vi "Select File.vi"(5 "PREV":bool, 6 "t in":i32, 7 "Bool Refnum in":refnum<vi>, 8 "error in (no error)":errorcluster, 9 "NEXT":bool, 10 "Bool Refnum 3":refnum<vi>, 11 "Boolean in":refnum<vi>) -> (0 "error out":errorcluster, 3 "t out":i32)   [LabVIEW 2020]
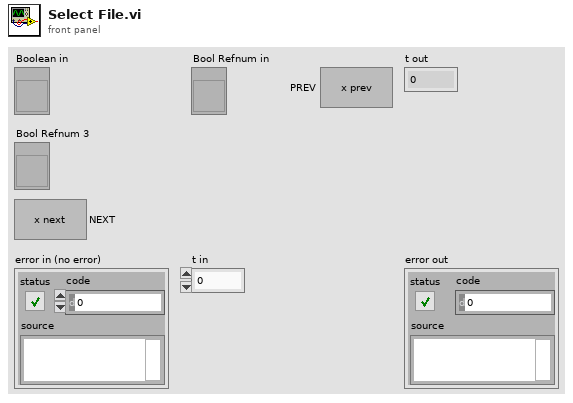
[diagram p1: front panel]
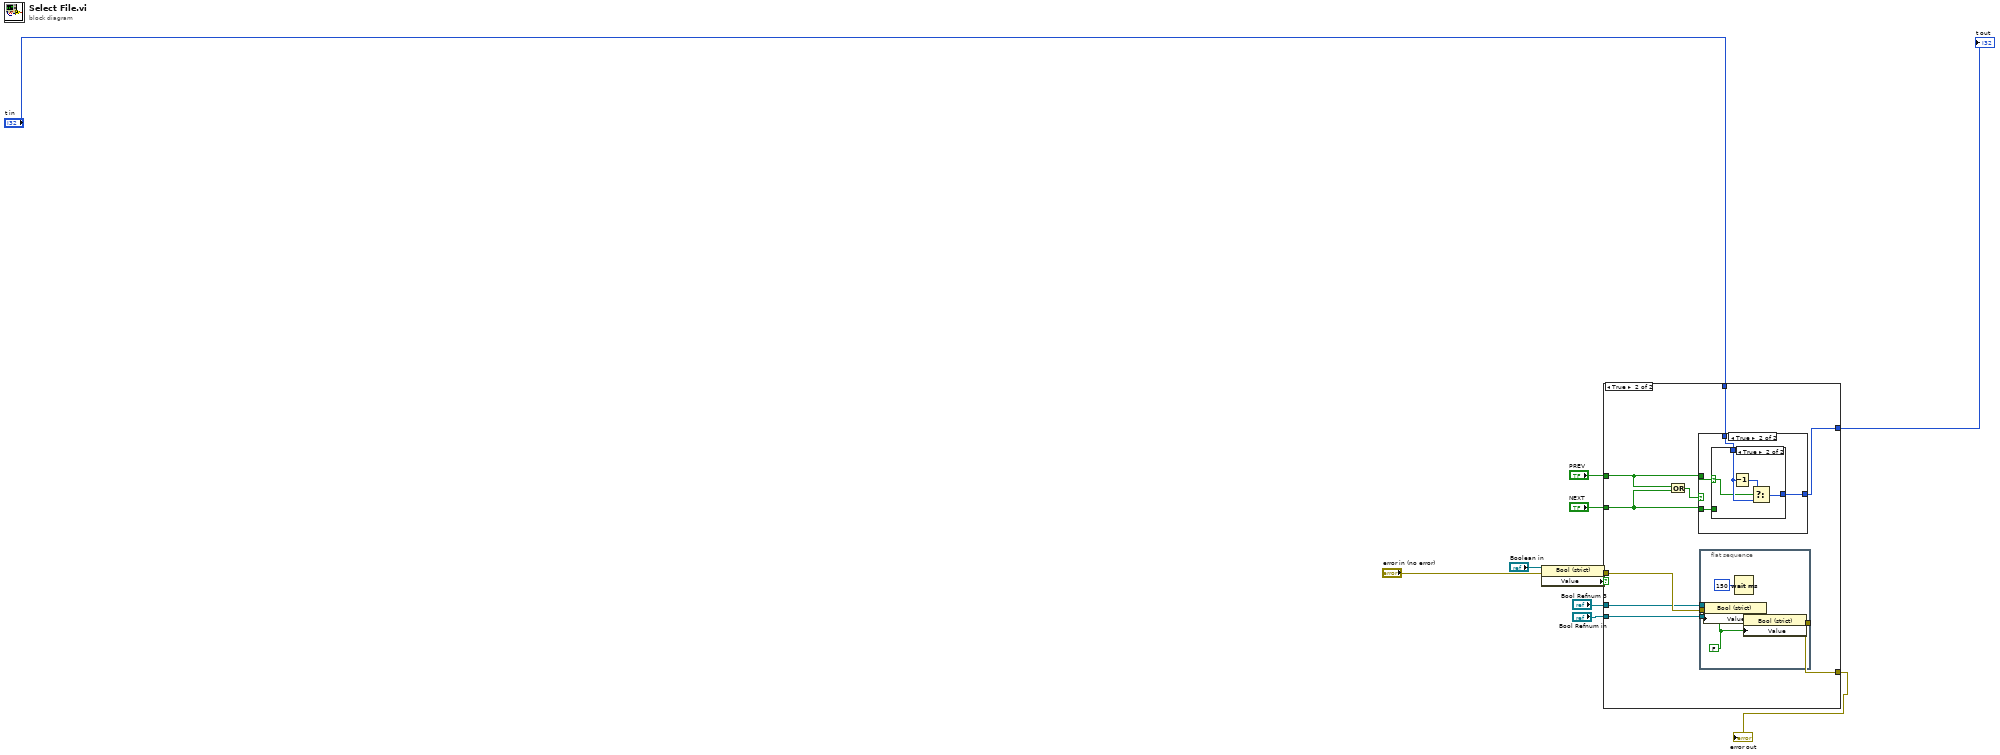
[diagram p0: block diagram]
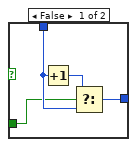
[diagram p4: hidden frame]
diagram:
  n1 = property on="Property Node" class="Bool (strict)"(reference="Boolean in", error in="error in (no error)") -> (error out=w9:errorcluster, "Value"=w6:bool)  [unwired: 1 out]
  n2 = case shown="True" w6 {
    tunnel: [w12 w22] -> w7
    tunnel: [w13 w21] -> w4
    tunnel: "t in" -> [w13 w20]
    tunnel: w9 -> [w12 w18]
    tunnel: "NEXT" -> [_ w17]
    tunnel: "PREV" -> [_ w16]
    tunnel: "Bool Refnum in" -> [_ w15]
    tunnel: "Bool Refnum 3" -> [_ w14]
    frame False {
    }
    frame True {
      n3 = Or(x=w16, y=w17) -> (x .or. y?=w19:bool)
      n4 = case shown="True" w19 {
        tunnel: [w30 w34] -> w21
        tunnel: w20 -> [w30 w33]
        tunnel: w16 -> [_ w32]
        tunnel: w17 -> [_ w31]
        frame False {
        }
        frame True {
          n5 = case shown="True" w32 {
            selector: w32 -> [_ w39]
            tunnel: [w38 w42] -> w34
            tunnel: w33 -> [w37 w41]
            tunnel: w31 -> [w35 _]
            frame False {
              n6 = Increment(x=w37) -> (x+1=w36:i32)
              n7 = Select(t=w36, s=w35, f=w37) -> (s? t:f=w38:i32)
            }
            frame True {
              n8 = Decrement(x=w41) -> (x-1=w40:i32)
              n9 = Select(t=w40, s=w39, f=w41) -> (s? t:f=w42:i32)
            }
          }
        }
      }
      n10 = flat-sequence {
        tunnel: w18 -> [w27]
        tunnel: [w29] -> w22
        tunnel: w15 -> [w24]
        tunnel: w14 -> [w23]
        frame #0 {
          w26 = FALSE ("NEXT")
          n11 = property on="Property Node" class="Bool (strict)"(reference=w23, error in=w27, "Value"=w26) -> (error out=w25:errorcluster)  [unwired: 1 out]
          n12 = Wait (ms)(milliseconds to wait=u32 150) -> ()  [unwired: 1 out]
          n13 = property on="Property Node" class="Bool (strict)"(reference=w24, error in=w25, "Value"=w26) -> (error out=w29:errorcluster)  [unwired: 1 out]
        }
      }
    }
  }
  "error out" <- w7
  "t out" <- w4
